vi "Write to Log Buffer.vi"(1 "error in":errorcluster, 2 "array of values":dbl[](array[numeric])=[0.0, 0.0, 0.0, 0.0, 0.0, 0.0, 0.0]) -> (0 "error out":errorcluster)   [LabVIEW 2016]
uses:
  Refname/Queues.ctl
  Main/Robot Global Data.vi
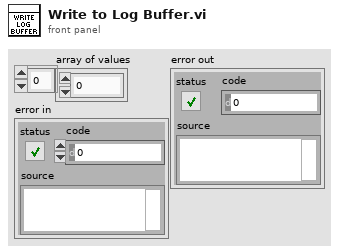
[diagram p1: front panel]
types:
  T1 = typedef "Queues.ctl" = enum16{"Log Queue"}
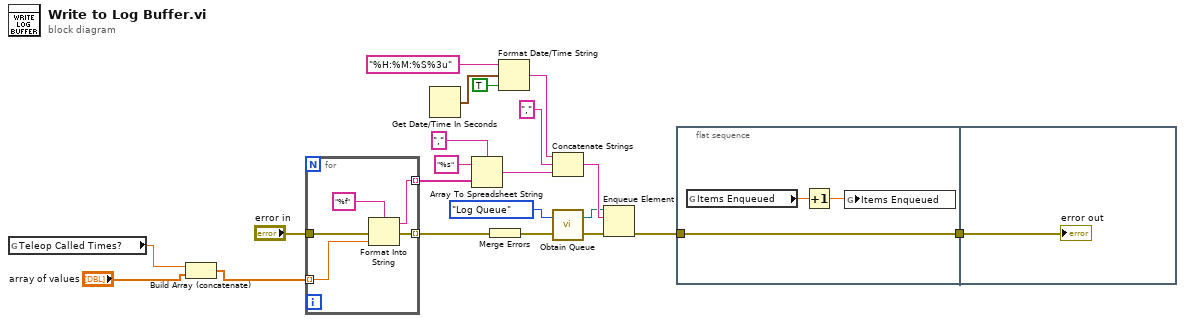
[diagram p0: block diagram]
diagram:
  n1 = global read "Robot Global Data.vi" "Teleop Called Times?"() -> (w2:dbl)
  n2 = Build Array (concatenate)(w2, "array of values") -> (w1:dbl[])
  n3 = for {
    tunnel: w1 -> [w26] mode=indexing
    tunnel: [w24] -> w20 mode=indexing
    tunnel: "error in" -> [w23]
    tunnel: [w22] -> w14 mode=indexing
    n4 = Format Into String(format string="%f", error in=w23, w26) -> (resulting string=w24:string, error out=w22:errorcluster)  [unwired: 1 in]
  }
  n5 = Get Date/Time In Seconds() -> (seconds since 1Jan1904=w7:timestamp)
  n6 = Array To Spreadsheet String(delimiter (Tab)=",", array=w20, 3:"%s" ("format string")) -> (spreadsheet string=w18:string)
  n7 = Merge Errors(w14) -> (w10:errorcluster)
  n8 = Format Date/Time String(time format string (%c)="%H:%M:%S%3u", seconds (now)=w7, UTC format=TRUE) -> (date/time string=w4:string)
  n9 = Concatenate Strings(w4, "," ("string"), w18) -> (w16:string)
  n10 = call "Obtain Queue.vi"("error in"=w10, "Queue"=Queues."Log Queue") -> ("error out"=w11:errorcluster, "Queue Ref"=w12:refnum<queue>)
  n11 = Enqueue Element(queue=w12, element=w16, error in (no error)=w11) -> (error out=w9:errorcluster)  [unwired: 1 in, 2 out]
  n12 = flat-sequence {
    tunnel: w9 -> [w29]
    tunnel: [w29] -> w8
    tunnel: w8 -> [w30]
    frame #0 {
      n13 = global read "Robot Global Data.vi" "Items Enqueued"() -> (w28:dbl)
      n14 = Increment(x=w28) -> (x+1=w27:dbl)
      n15 = global write "Robot Global Data.vi" "Items Enqueued"(w27) -> ()
    }
    frame #1 {
      "error out" <- w30
    }
  }
